vi "PSVCH_Formula Edit.vi"(8 "error in":errorcluster, 9 "Symbol Path":path, 10 "UsedChList[]":T2(array[cluster]), 11 "Formula In":string) -> (0 "Error Out":errorcluster, 2 "Formula":string, 3 "Cancel?":bool)   [LabVIEW 2016]
uses:
  <vilib>/Utility/error.llb/DialogType.ctl
  <vilib>/express/express arith-compare/Formula/XNode/ExpressFormulaBlockNode.xnode
panel:
  in  "Data Source":string(tree)
  in  "Formula":string caption="信号处理"
  out "Error":string caption="错误信息"
  in  "Calculator":T1 caption="计算器"
  in  "Cancel":bool
  in  "OK":bool
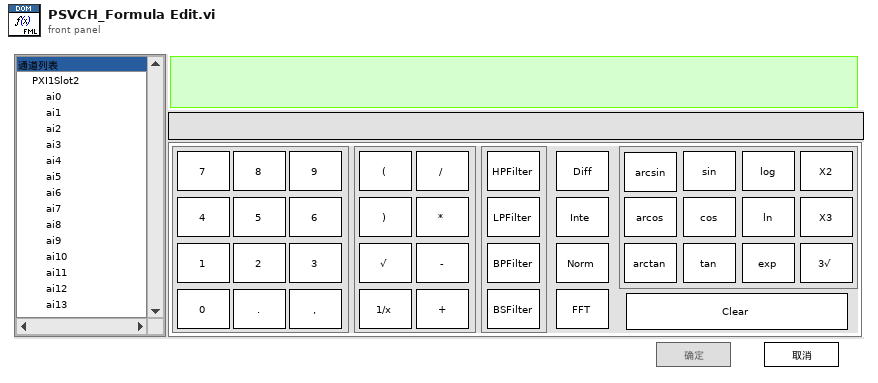
[diagram p1: front panel]
types:
  T1 = cluster{"Cal_0":bool, "Cal_1":bool, "Cal_2":bool, "Cal_3":bool, "Cal_4":bool, "Cal_5":bool, "Cal_6":bool, "Cal_7":bool, "Cal_8":bool, "Cal_9":bool, "Cal_+":bool, "Cal_-":bool, "Cal_*":bool, "Cal_/":bool, "Cal_sin":bool, "Cal_cos":bool, "Cal_diff":bool, "Cal_inte":bool, "Cal_Clear":bool, "Cal_.":bool, "Cal_(":bool, "Cal_)":bool, "Cal_fft":bool, "Cal_,":bool, "Cal_BSFilter":bool, "Cal_BPFilter":bool, "Cal_LPFilter":bool, "Cal_Reciprocal":bool, "Cal_HPFilter":bool, "Cal_Normalize":bool, "Cal_√":bool, "Cal_sinh":bool, "Cal_cosh":bool, "Cal_tan":bool, "Cal_Tanh":bool, "Cal_log":bool, "Cal_ln":bool, "Cal_exp":bool, "Cal_X2":bool, "Cal_X3":bool, "Cal_3√":bool}
  T2 = cluster{"ModuTag":string, "ModuAlias":string, "ChanTag[]":string[], "ChanAlias[]":string[], "ChanUnit[]":string[]}[]
  T3 = cluster{"Error":errorcluster, "Exit":bool, "Cancel?":bool, "Ref":cluster{"Formula":refnum<vi>, "OK":refnum<vi>, "Error":refnum<vi>, "Data Source":refnum<vi>}, "Formula":string, "VarList":cluster{"Tag":string[], "Name":string[]}, "Symbol Path":path, "UsedChList[]":cluster{"ModuTag":string, "ModuAlias":string, "ChanTag[]":string[], "ChanAlias[]":string[], "ChanUnit[]":string[]}[]}
  T4 = enum8{"Enabled", "Disabled", "Disabled and Grayed Out"}
  T5 = typedef "LVPoint32TypeDef.ctl" = cluster{"Horizontal":i32, "Vertical":i32}
  T6 = cluster{"data name":string, "drag data":variant}[]
  T7 = typedef "DialogType.ctl" = u16
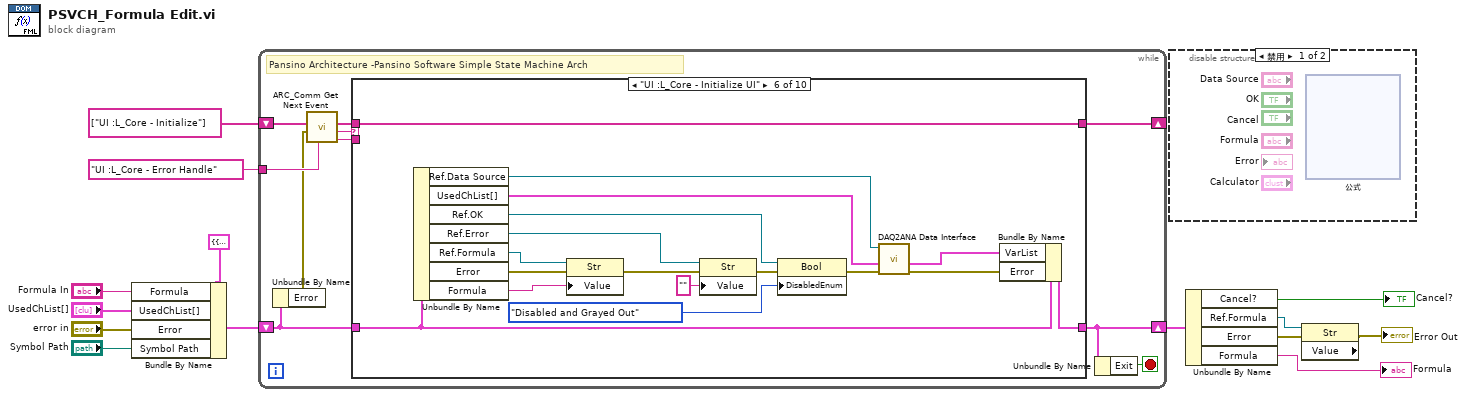
[diagram p0: block diagram]
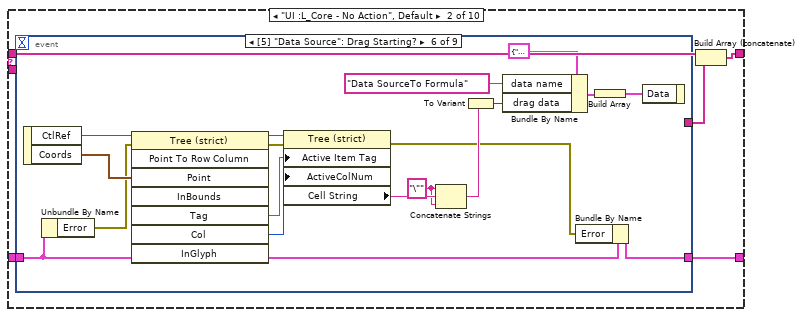
[diagram p3: hidden frame]
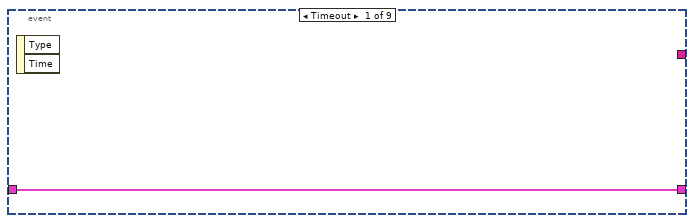
[diagram p4: hidden frame]
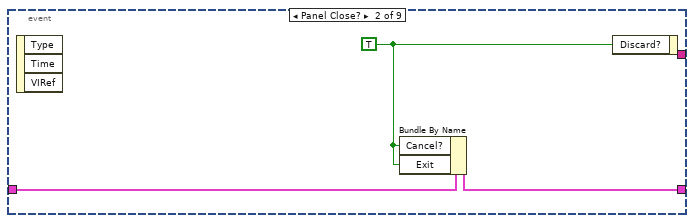
[diagram p5: hidden frame]
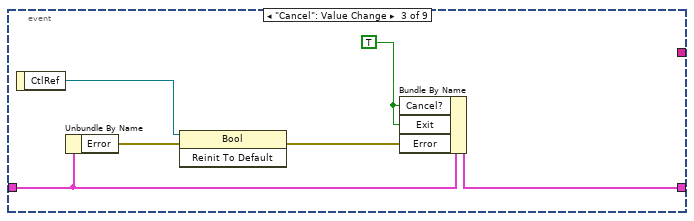
[diagram p6: hidden frame]
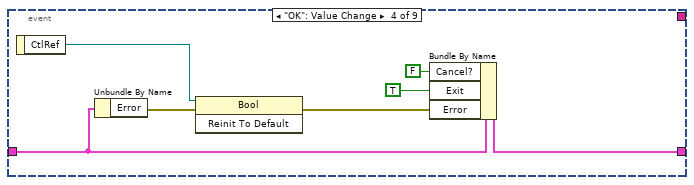
[diagram p7: hidden frame]
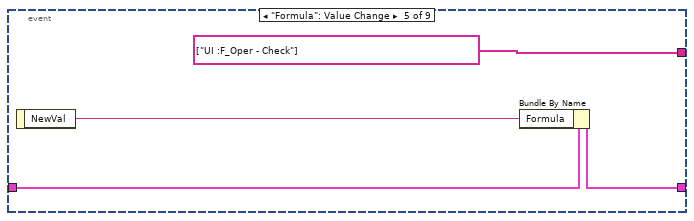
[diagram p8: hidden frame]
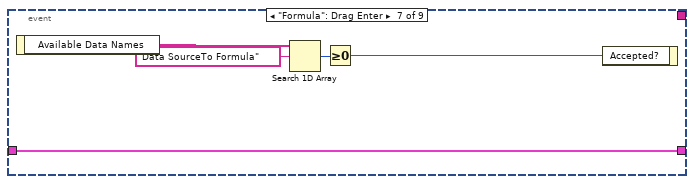
[diagram p9: hidden frame]
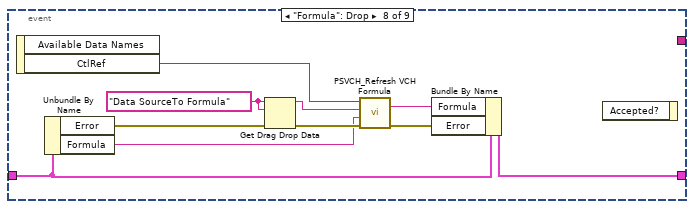
[diagram p10: hidden frame]
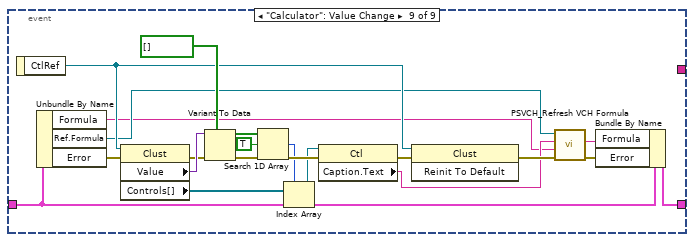
[diagram p11: hidden frame]
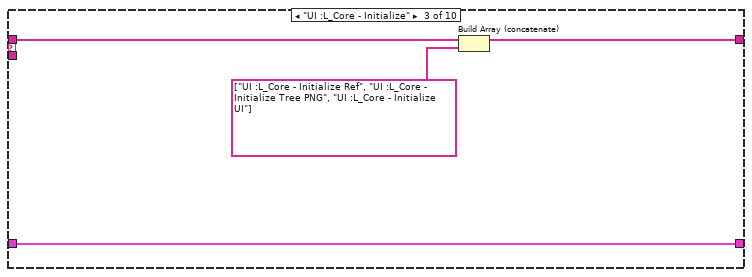
[diagram p12: hidden frame]
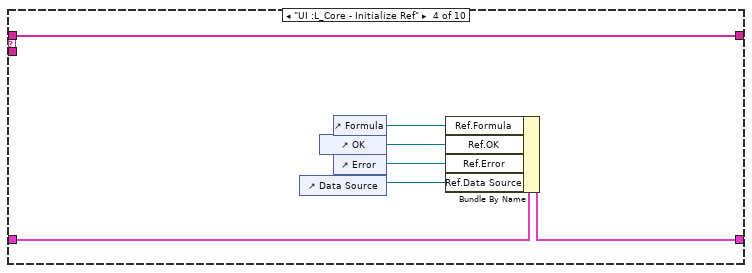
[diagram p13: hidden frame]
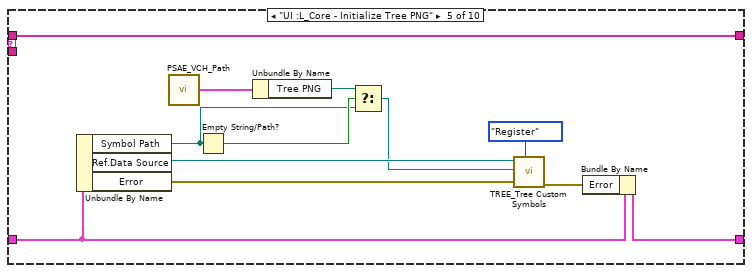
[diagram p14: hidden frame]
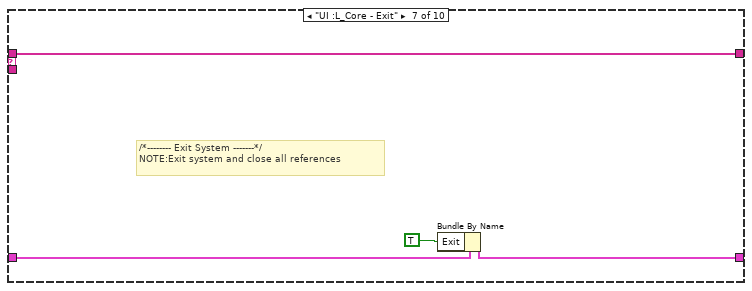
[diagram p15: hidden frame]
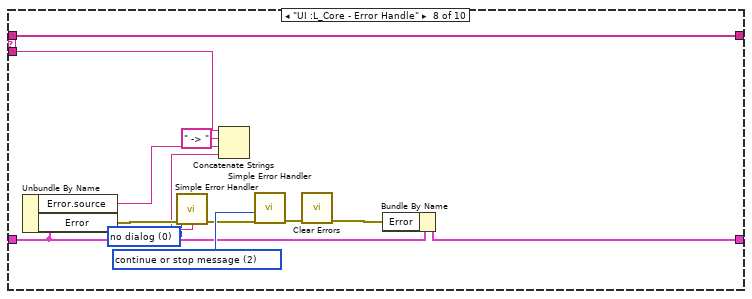
[diagram p16: hidden frame]
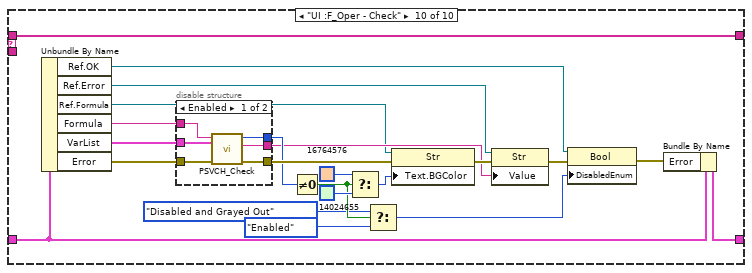
[diagram p18: hidden frame]
diagram:
  n1 = Bundle By Name(cluster=T3 {"Error"={"status"=FALSE, "code"=0, "source"=""}, "Exit"=FALSE, "Cancel?"=FALSE, "Ref"={"Formula"=refnum, "OK"=refnum, "Error"=refnum, "Data Source"=refnum}, "Formula"="", "VarList"={"Tag"=[], "Name"=[]}, "Symbol Path"=path "", "UsedChList[]"=[]} ("Temp Variable"), "Formula"="Formula In", "UsedChList[]"="UsedChList[]", "Error"="error in", "Symbol Path"="Symbol Path") -> (w7:T3)
  n2 = while {
    tunnel: "UI :L_Core - Error Handle" ("Error Handle") -> [w23]
    shift-right: [w21] -> _
    shift-left: string[] ["UI :L_Core - Initialize"] -> [w24]
    shift-right: [w18] -> w11
    shift-left: w7 -> [w20]
    stop <- w17 stop-if-true
    # "Pansino Architecture -Pansino Software Simple State Machine Arch"
    n3 = Unbundle By Name(w20) -> ("Error"=w19:errorcluster)
    n4 = call "ARC_Comm Get Next Event.vi"("Error Handle"=w23, "error in (no error)"=w19, "event queue in"=w24) -> ("prev event"=w15:string, "next event"=w16:string, "event queue out"=w22:string[])  [unwired: 3 in]
    n5 = case shown="\"UI :L_Core - Initialize UI\"" w16 {
      tunnel: w22 -> [w26 w31 w109 w116 w128 w145 w149 w162 w164 w186]
      tunnel: [w26 w30 w107 w116 w128 w145 w149 w162 w164 w186] -> w21
      tunnel: w20 -> [w25 w29 w108 w115 w125 w144 w148 w159 w163 w185]
      tunnel: [w25 w28 w108 w114 w123 w139 w147 w158 w163 w184] -> w18
      tunnel: w15 -> [_ _ _ _ _ _ _ w151 _ _]
      frame "----------Core Status----------" {
      }
      frame "UI :L_Core - No Action", Default {
        n6 = event shown="[5] \"Data Source\": Drag Starting?" {
          selector: _ -> [_ _ _ _ _ _ _ _ _]
          dyn-events: _ -> [_ _ _ _ _ _ _ _ _]
          timeout: _ -> [_ _ _ _ _ _ _ _ _]
          tunnel: w29 -> [w32 w35 w38 w43 w52 w68 w72 w85 w105]
          tunnel: [w32 w34 w41 w48 w50 w61 w72 w81 w91] -> w28
          tunnel: [_ _ _ _ string[] ["UI :F_Oper - Check"] ("数组") _ _ _ _] -> w27
          event Timeout {
            n7 = event-data() -> ()  [unwired: 1 in, 2 out]
          }
          event Panel Close? {
            w33 = TRUE ("放弃？")
            n8 = event-data() -> ()  [unwired: 1 in, 3 out]
            n9 = Bundle By Name(cluster=w35, "Cancel?"=w33, "Exit"=w33) -> (w34:T3)
            n10 = event-data("Discard?"=w33) -> ()  [unwired: 1 in, 1 out]
          }
          event "Cancel": Value Change {
            w40 = TRUE ("放弃？")
            n11 = event-data() -> ("CtlRef"=w36:refnum<vi>)  [unwired: 1 in]
            n12 = Unbundle By Name(w38) -> ("Error"=w37:errorcluster)
            n13 = invoke class="Bool" method="Reinit To Default"(reference=w36, error in=w37) -> (error out=w39:errorcluster)  [unwired: 1 in, 2 out]
            n14 = Bundle By Name(cluster=w38, "Cancel?"=w40, "Exit"=w40, "Error"=w39) -> (w41:T3)
          }
          event "OK": Value Change {
            n15 = event-data() -> ("CtlRef"=w44:refnum<vi>)  [unwired: 1 in]
            n16 = Unbundle By Name(w43) -> ("Error"=w42:errorcluster)
            n17 = invoke class="Bool" method="Reinit To Default"(reference=w44, error in=w42) -> (error out=w45:errorcluster)  [unwired: 1 in, 2 out]
            n18 = Bundle By Name(cluster=w43, "Cancel?"=FALSE, "Exit"=TRUE, "Error"=w45) -> (w48:T3)
          }
          event "Formula": Value Change {
            n19 = event-data() -> ("NewVal"=w49:string)  [unwired: 1 in]
            n20 = Bundle By Name(cluster=w52, "Formula"=w49) -> (w50:T3)
          }
          event "Data Source": Drag Starting? {
            w55 = "\"" ("字符串")
            n21 = event-data() -> ("CtlRef"=w70:refnum<vi>, "Coords"=w69:T5)  [unwired: 1 in]
            n22 = Unbundle By Name(w68) -> ("Error"=w67:errorcluster)
            n23 = invoke class="Tree (strict)" method="Point To Row Column"(reference=w70, error in=w67, "Point"=w69) -> (reference out=w60:refnum<vi>, error out=w59:errorcluster, "Tag"=w58:string, "Col"=w57:i32)  [unwired: 5 in, 4 out]
            n24 = property class="Tree (strict)"(reference=w60, error in=w59, "Active Item Tag"=w58, "ActiveColNum"=w57) -> (error out=w53:errorcluster, "Cell String"=w56:string)  [unwired: 1 out]
            n25 = Concatenate Strings(w55, w56, w55) -> (w54:string)
            n26 = To Variant(anything=w54) -> (Variant=w64:variant)
            n27 = Bundle By Name(cluster=cluster{"data name":string, "drag data":variant} {"data name"="", "drag data"=variant}, "data name"="Data SourceTo Formula" ("元素"), "drag data"=w64) -> (w63:cluster{"data name":string, "drag data":variant})
            n28 = Bundle By Name(cluster=w68, "Error"=w53) -> (w61:T3)
            n29 = Build Array(w63) -> (w62:T6)
            n30 = event-data("Data"=w62) -> ()  [unwired: 1 in, 1 out]
          }
          event "Formula": Drag Enter {
            n31 = event-data() -> ("Available Data Names"=w74:string[])  [unwired: 1 in]
            n32 = Search 1D Array(1D array=w74, element="Data SourceTo Formula" ("元素")) -> (index of element=w75:i32)  [unwired: 1 in]
            n33 = Greater Or Equal To 0?(x=w75) -> (x >= 0?=w73:bool)
            n34 = event-data("Accepted?"=w73) -> ()  [unwired: 1 in, 1 out]
          }
          event "Formula": Drop {
            w83 = "Data SourceTo Formula" ("元素")
            n35 = event-data() -> ("CtlRef"=w78:refnum<vi>)  [unwired: 1 in, 1 out]
            n36 = Unbundle By Name(w85) -> ("Error"=w84:errorcluster, "Formula"=w76:string)
            n37 = Get Drag Drop Data(6:w84, 8:w83, 9:w83) -> (0:w82:errorcluster, 3:w79:string)
            n38 = call "PSVCH_Refresh VCH Formula.vi"("error in"=w82, "Formula In"=w76, "String"=w79, "Ref.Formula"=w78) -> ("error out"=w80:errorcluster, "result string"=w77:string)  [unwired: 6 in]
            n39 = Bundle By Name(cluster=w85, "Formula"=w77, "Error"=w80) -> (w81:T3)
            n40 = event-data() -> ()  [unwired: 2 in, 1 out]
          }
          event "Calculator": Value Change {
            n41 = event-data() -> ("CtlRef"=w93:refnum<vi>)  [unwired: 1 in]
            n42 = Unbundle By Name(w105) -> ("Formula"=w86:string, "Ref.Formula"=w87:refnum<vi>, "Error"=w104:errorcluster)
            n43 = property class="Clust"(reference=w93, error in=w104) -> (error out=w102:errorcluster, "Value"=w103:variant, "Controls[]"=w97:refnum<vi>[])  [unwired: 1 out]
            n44 = Variant To Data(error in=w102, type=bool[] [], Variant=w103) -> (data=w100:bool[], error out=w98:errorcluster)
            n45 = Search 1D Array(1D array=w100, element=TRUE) -> (index of element=w96:i32)  [unwired: 1 in]
            n46 = Index Array(array=w97, index=w96) -> (element=w95:refnum<vi>)
            n47 = property class="Ctl"(reference=w95, error in=w98) -> (error out=w94:errorcluster, "Caption.Text"=w88:string)  [unwired: 1 out]
            n48 = invoke class="Clust" method="Reinit To Default"(reference=w93, error in=w94) -> (error out=w92:errorcluster)  [unwired: 1 in, 2 out]
            n49 = call "PSVCH_Refresh VCH Formula.vi"("error in"=w92, "Formula In"=w86, "String"=w88, "Ref.Formula"=w87) -> ("error out"=w90:errorcluster, "result string"=w89:string)  [unwired: 6 in]
            n50 = Bundle By Name(cluster=w105, "Formula"=w89, "Error"=w90) -> (w91:T3)
          }
        }
        n51 = Build Array (concatenate)(w31, w27) -> (w30:string[])
      }
      frame "UI :L_Core - Initialize" {
        n52 = Build Array (concatenate)(w109, string[] ["UI :L_Core - Initialize Ref", "UI :L_Core - Initialize Tree PNG", "UI :L_Core - Initialize UI"] ("数组")) -> (w107:string[])
      }
      frame "UI :L_Core - Initialize Ref" {
        n53 = control-ref of="Data Source"() -> (w111:refnum<vi>)
        n54 = control-ref of="OK"() -> (w113:refnum<vi>)
        n55 = control-ref of="Formula"() -> (w110:refnum<vi>)
        n56 = control-ref of="Error"() -> (w112:refnum<vi>)
        n57 = Bundle By Name(cluster=w115, "Ref.Formula"=w110, "Ref.OK"=w113, "Ref.Error"=w112, "Ref.Data Source"=w111) -> (w114:T3)
      }
      frame "UI :L_Core - Initialize Tree PNG" {
        n58 = Unbundle By Name(w125) -> ("Symbol Path"=w120:path, "Ref.Data Source"=w126:refnum<vi>, "Error"=w127:errorcluster)
        n59 = call "PSAE_VCH_Path.vi"() -> ("All Path"=w119:cluster{"Tree PNG":path, "Data":path})  [unwired: 11 in]
        n60 = Empty String/Path?(string/path=w120) -> (empty?=w121:bool)
        n61 = Unbundle By Name(w119) -> ("Tree PNG"=w118:path)
        n62 = Select(t=w118, s=w121, f=w120) -> (s? t:f=w117:path)
        n63 = call "TREE_Tree Custom Symbols.vi"("Operation"=enum16{"Register", "GetIndex"}."Register", "error in"=w127, "Files"=w117, "tree refnum"=w126) -> ("error out"=w124:errorcluster)  [unwired: 6 in, 1 out]
        n64 = Bundle By Name(cluster=w125, "Error"=w124) -> (w123:T3)
      }
      frame "UI :L_Core - Initialize UI" {
        n65 = Unbundle By Name(w144) -> ("Ref.Data Source"=w135:refnum<vi>, "UsedChList[]"=w129:T2, "Ref.OK"=w141:refnum<vi>, "Ref.Error"=w132:refnum<vi>, "Ref.Formula"=w143:refnum<vi>, "Error"=w142:errorcluster, "Formula"=w138:string)
        n66 = property class="Str"(reference=w143, error in=w142, "Value"=w138) -> (error out=w134:errorcluster)  [unwired: 1 out]
        n67 = property class="Str"(reference=w132, error in=w134, "Value"="") -> (error out=w133:errorcluster)  [unwired: 1 out]
        n68 = property class="Bool"(reference=w141, error in=w133, "DisabledEnum"=T4."Disabled and Grayed Out" ("禁用")) -> (error out=w137:errorcluster)  [unwired: 1 out]
        n69 = call "DAQ2ANA Data Interface.vi"("error in"=w137, "UsedChList[]"=w129, "Tree Ref"=w135) -> ("error out"=w136:errorcluster, "VariList"=w130:cluster{"Tag[]":string[], "Name[]":string[]})  [unwired: 7 in]
        n70 = Bundle By Name(cluster=w144, "VarList"=w130, "Error"=w136) -> (w139:T3)
      }
      frame "UI :L_Core - Exit" {
        # "/*-------- Exit System -------*/\nNOTE:Exit system and close all references"
        n71 = Bundle By Name(cluster=w148, "Exit"=TRUE) -> (w147:T3)
      }
      frame "UI :L_Core - Error Handle" {
        w150 = T7 0 items=["no dialog", "OK message", "continue or stop message", "OK message + warnings", "continue/stop + warnings"] ("type of dialog (OK msg:1)")
        w161 = T7 2 items=["no dialog", "OK message", "continue or stop message", "OK message + warnings", "continue/stop + warnings"] ("type of dialog (OK msg:1)")
        n72 = Unbundle By Name(w159) -> ("Error.source"=w155:string, "Error"=w156:errorcluster)
        n73 = call <vilib>:"Simple Error Handler.vi"("type of dialog (OK msg:1)"=w150, "error in (no error)"=w156) -> ("error out"=w154:errorcluster, "message"=w153:string)  [unwired: 3 in, 3 out]
        n74 = Concatenate Strings(w151, " -> " ("字符串"), w155, w153) -> ()  [unwired: 1 out]
        n75 = call <vilib>:"Simple Error Handler.vi"("type of dialog (OK msg:1)"=w161, "error in (no error)"=w154) -> ("error out"=w160:errorcluster)  [unwired: 3 in, 4 out]
        n76 = call <vilib>:"Clear Errors.vi"("error in (no error)"=w160) -> ("error out"=w157:errorcluster)  [unwired: 5 in, 1 out]
        n77 = Bundle By Name(cluster=w159, "Error"=w157) -> (w158:T3)
      }
      frame "----------Operation----------" {
      }
      frame "UI :F_Oper - Check" {
        n78 = Unbundle By Name(w185) -> ("Ref.OK"=w174:refnum<vi>, "Ref.Error"=w177:refnum<vi>, "Ref.Formula"=w166:refnum<vi>, "Formula"=w165:string, "VarList"=w168:cluster{"Tag":string[], "Name":string[]}, "Error"=w167:errorcluster)
        n79 = disable-structure shown="Enabled" {
          disable-tunnel: [w192 w193] -> w180
          disable-tunnel: [w191 _] -> w179
          disable-tunnel: [w190 _] -> w176
          disable-tunnel: w168 -> [w189 _]
          disable-tunnel: w167 -> [w188 w193]
          disable-tunnel: w165 -> [w187 _]
          frame Enabled {
            n80 = call "PSVCH_Check.vi"("Error In (no error)"=w188, "VarList"=w189, "Formula"=w187) -> ("Error Out"=w192:errorcluster, "source"=w190:string, "code"=w191:i32)  [unwired: 4 in, 2 out]
          }
          frame Disabled {
          }
        }
        n81 = Not Equal To 0?(x=w179) -> (x != 0?=w171:bool)
        n82 = Select(t=u32 16764576 ("Color 2"), s=w171, f=u32 14024655 ("Color")) -> (s? t:f=w181:u32)
        n83 = Select(t=T4."Disabled and Grayed Out", s=w171, f=T4."Enabled" ("禁用")) -> (s? t:f=w169:T4)
        n84 = property class="Str"(reference=w166, error in=w180, "Text.BGColor"=w181) -> (error out=w178:errorcluster)  [unwired: 1 out]
        n85 = property class="Str"(reference=w177, error in=w178, "Value"=w176) -> (error out=w175:errorcluster)  [unwired: 1 out]
        n86 = property class="Bool"(reference=w174, error in=w175, "DisabledEnum"=w169) -> (error out=w173:errorcluster)  [unwired: 1 out]
        n87 = Bundle By Name(cluster=w185, "Error"=w173) -> (w184:T3)
      }
    }
    n88 = Unbundle By Name(w18) -> ("Exit"=w17:bool)
  }
  n89 = disable-structure shown="禁用" {
    frame Disabled {
      n90 = xnode "公式"() -> ()  [unwired: 2 in, 2 out]
    }
    frame Enabled {
    }
  }
  n91 = Unbundle By Name(w11) -> ("Cancel?"=→"Cancel?":bool, "Ref.Formula"=w9:refnum<vi>, "Error"=w8:errorcluster, "Formula"=→"Formula":string)
  n92 = property class="Str" props=["Value"](reference=w9, error in=w8) -> (error out=→"Error Out":errorcluster)  [unwired: 2 out]
